vi "Dresden Edit Recipe(in).vi"() -> ()   [LabVIEW 2009] (continued)
                    n653 = local read "R Single DC Step9 Coating Power"() -> (w1514:dbl)
                    n654 = local read "R Single DC Interval length9"() -> (w1513:dbl)
                    n655 = Equal To 0?(x=w1514) -> (x = 0?=w1516:bool)
                    n656 = Equal To 0?(x=w1513) -> (x = 0?=w1515:bool)
                  }
                }
                n657 = case shown="True" w1333 {
                  tunnel: [FALSE w1654] -> w1271
                  tunnel: [FALSE w1651] -> w1270
                  frame #0 {
                  }
                  frame #1 {
                    # "15"
                    # "14"
                    n658 = local read "R Single DC Step4 Coating Power"() -> (w1653:dbl)
                    n659 = local read "R Single DC Interval length4"() -> (w1652:dbl)
                    n660 = Equal To 0?(x=w1653) -> (x = 0?=w1654:bool)
                    n661 = Equal To 0?(x=w1652) -> (x = 0?=w1651:bool)
                  }
                }
                n662 = case shown="True" w1302 {
                  tunnel: [FALSE w1533] -> w1267
                  tunnel: [FALSE w1531] -> w1266
                  frame #0 {
                  }
                  frame #1 {
                    # "19"
                    # "18"
                    n663 = local read "R Single DC Step6 Coating Power"() -> (w1534:dbl)
                    n664 = local read "R Single DC Interval length6"() -> (w1532:dbl)
                    n665 = Equal To 0?(x=w1534) -> (x = 0?=w1533:bool)
                    n666 = Equal To 0?(x=w1532) -> (x = 0?=w1531:bool)
                  }
                }
                n667 = case shown="True" w1326 {
                  tunnel: [FALSE w1628] -> w1251
                  tunnel: [FALSE w1625] -> w1250
                  frame #0 {
                  }
                  frame #1 {
                    # "32"
                    # "31"
                    n668 = local read "R Single RF  Step1 Coating Power"() -> (w1627:dbl)
                    n669 = local read "R Single RF Interval length"() -> (w1626:dbl)
                    n670 = Equal To 0?(x=w1626) -> (x = 0?=w1625:bool)
                    n671 = Equal To 0?(x=w1627) -> (x = 0?=w1628:bool)
                  }
                }
                n672 = case shown="True" w1325 {
                  tunnel: [FALSE w1622] -> w1249
                  tunnel: [FALSE w1619] -> w1248
                  frame #0 {
                  }
                  frame #1 {
                    # "34"
                    # "33"
                    n673 = local read "R Single RF Step2 Coating Power"() -> (w1621:dbl)
                    n674 = local read "R Single RF Interval length2"() -> (w1620:dbl)
                    n675 = Equal To 0?(x=w1621) -> (x = 0?=w1622:bool)
                    n676 = Equal To 0?(x=w1620) -> (x = 0?=w1619:bool)
                  }
                }
                n677 = case shown="True" w1308 {
                  tunnel: [FALSE w1610] -> w1245
                  tunnel: [FALSE w1607] -> w1244
                  frame #0 {
                  }
                  frame #1 {
                    # "38"
                    # "37"
                    n678 = local read "R Single RF Step4 Coating Power"() -> (w1609:dbl)
                    n679 = local read "R Single RF Interval length4"() -> (w1608:dbl)
                    n680 = Equal To 0?(x=w1609) -> (x = 0?=w1610:bool)
                    n681 = Equal To 0?(x=w1608) -> (x = 0?=w1607:bool)
                  }
                }
                n682 = case shown="True" w1298 {
                  tunnel: [FALSE w1502] -> w1241
                  tunnel: [FALSE w1501] -> w1240
                  frame #0 {
                  }
                  frame #1 {
                    # "42"
                    # "41"
                    n683 = local read "R Single RF Step6 Coating Power"() -> (w1504:dbl)
                    n684 = local read "R Single RF Interval length6"() -> (w1503:dbl)
                    n685 = Equal To 0?(x=w1504) -> (x = 0?=w1502:bool)
                    n686 = Equal To 0?(x=w1503) -> (x = 0?=w1501:bool)
                  }
                }
                n687 = case shown="True" w1297 {
                  tunnel: [FALSE w1496] -> w1239
                  tunnel: [FALSE w1495] -> w1237
                  frame #0 {
                  }
                  frame #1 {
                    # "44"
                    # "43"
                    n688 = local read "R Single RF Step7 Coating Power"() -> (w1498:dbl)
                    n689 = local read "R Single RF Interval length7"() -> (w1497:dbl)
                    n690 = Equal To 0?(x=w1498) -> (x = 0?=w1496:bool)
                    n691 = Equal To 0?(x=w1497) -> (x = 0?=w1495:bool)
                  }
                }
                n692 = case shown="True" w1296 {
                  tunnel: [FALSE w1490] -> w1238
                  tunnel: [FALSE w1489] -> _
                  frame #0 {
                  }
                  frame #1 {
                    # "46"
                    # "45"
                    n693 = local read "R Single RF Step8 Coating Power"() -> (w1492:dbl)
                    n694 = local read "R Single RF Interval length8"() -> (w1491:dbl)
                    n695 = Equal To 0?(x=w1492) -> (x = 0?=w1490:bool)
                    n696 = Equal To 0?(x=w1491) -> (x = 0?=w1489:bool)
                  }
                }
                n697 = case shown="True" w1336 {
                  tunnel: [FALSE w1672] -> w1277
                  tunnel: [FALSE w1669] -> w1276
                  frame #0 {
                  }
                  frame #1 {
                    # "9"
                    # "8"
                    n698 = local read "R Single DC Step1 Coating Power"() -> (w1671:dbl)
                    n699 = local read "R Single DC Interval length1"() -> (w1670:dbl)
                    n700 = Equal To 0?(x=w1671) -> (x = 0?=w1672:bool)
                    n701 = Equal To 0?(x=w1670) -> (x = 0?=w1669:bool)
                  }
                }
                n702 = case shown="True" w1335 {
                  tunnel: [FALSE w1666] -> w1275
                  tunnel: [FALSE w1663] -> w1274
                  frame #0 {
                  }
                  frame #1 {
                    # "11"
                    # "10"
                    n703 = local read "R Single DC Step2 Coating Power"() -> (w1665:dbl)
                    n704 = local read "R Single DC Interval length2"() -> (w1664:dbl)
                    n705 = Equal To 0?(x=w1664) -> (x = 0?=w1663:bool)
                    n706 = Equal To 0?(x=w1665) -> (x = 0?=w1666:bool)
                  }
                }
                n707 = case shown="True" w1300 {
                  tunnel: [FALSE w1520] -> w1263
                  tunnel: [FALSE w1519] -> w1262
                  frame #0 {
                  }
                  frame #1 {
                    # "23"
                    # "22"
                    n708 = local read "R Single DC Step8 Coating Power"() -> (w1522:dbl)
                    n709 = local read "R Single DC Interval length8"() -> (w1521:dbl)
                    n710 = Equal To 0?(x=w1522) -> (x = 0?=w1520:bool)
                    n711 = Equal To 0?(x=w1521) -> (x = 0?=w1519:bool)
                  }
                }
                n712 = case shown="True" w1324 {
                  tunnel: [FALSE w1604] -> w1243
                  tunnel: [FALSE w1601] -> w1242
                  frame #0 {
                  }
                  frame #1 {
                    # "40"
                    # "39"
                    n713 = local read "R Single RF Step5 Coating Power"() -> (w1603:dbl)
                    n714 = local read "R Single RF Interval length5"() -> (w1602:dbl)
                    n715 = Equal To 0?(x=w1603) -> (x = 0?=w1604:bool)
                    n716 = Equal To 0?(x=w1602) -> (x = 0?=w1601:bool)
                  }
                }
                n717 = case shown="True" w1334 {
                  tunnel: [FALSE w1660] -> w1273
                  tunnel: [FALSE w1658] -> w1272
                  frame #0 {
                  }
                  frame #1 {
                    # "13"
                    # "12"
                    n718 = local read "R Single DC Step3 Coating Power"() -> (w1659:dbl)
                    n719 = local read "R Single DC Interval length3"() -> (w1657:dbl)
                    n720 = Equal To 0?(x=w1659) -> (x = 0?=w1660:bool)
                    n721 = Equal To 0?(x=w1657) -> (x = 0?=w1658:bool)
                  }
                }
                n722 = case shown="True" w1301 {
                  tunnel: [FALSE w1528] -> w1265
                  tunnel: [FALSE w1527] -> w1264
                  frame #0 {
                  }
                  frame #1 {
                    # "21"
                    # "20"
                    n723 = local read "R Single DC Step7 Coating Power"() -> (w1526:dbl)
                    n724 = local read "R Single DC Interval length7"() -> (w1525:dbl)
                    n725 = Equal To 0?(x=w1526) -> (x = 0?=w1528:bool)
                    n726 = Equal To 0?(x=w1525) -> (x = 0?=w1527:bool)
                  }
                }
                n727 = case shown="True" w1309 {
                  tunnel: [FALSE w1616] -> w1247
                  tunnel: [FALSE w1613] -> w1246
                  frame #0 {
                  }
                  frame #1 {
                    # "36"
                    # "35"
                    n728 = local read "R Single RF Step3 Coating Power"() -> (w1615:dbl)
                    n729 = local read "R Single RF Interval length3"() -> (w1614:dbl)
                    n730 = Equal To 0?(x=w1614) -> (x = 0?=w1613:bool)
                    n731 = Equal To 0?(x=w1615) -> (x = 0?=w1616:bool)
                  }
                }
                n732 = case shown="True" w1327 {
                  tunnel: [FALSE w1631] -> w1252
                  frame #0 {
                  }
                  frame #1 {
                    # "30"
                    n733 = local read "R Single RF Ramp up Time"() -> (w1630:dbl)
                    n734 = Equal To 0?(x=w1630) -> (x = 0?=w1631:bool)
                  }
                }
                n735 = case shown="True" w1179 {
                  tunnel: [FALSE w1508] -> w1259
                  tunnel: [FALSE w1507] -> w1258
                  frame #0 {
                  }
                  frame #1 {
                    # "27"
                    # "26"
                    n736 = local read "R Single DC Step10 Coating Power"() -> (w1510:dbl)
                    n737 = local read "R Single DC Interval length10"() -> (w1509:dbl)
                    n738 = Equal To 0?(x=w1510) -> (x = 0?=w1508:bool)
                    n739 = Equal To 0?(x=w1509) -> (x = 0?=w1507:bool)
                  }
                }
                n740 = case shown="True" w1331 {
                  tunnel: [FALSE w1638] -> w1257
                  tunnel: [FALSE w1634] -> w1256
                  frame #0 {
                  }
                  frame #1 {
                    # "29"
                    # "28"
                    n741 = local read "R Single RF Target material"() -> (w1636:string)
                    n742 = local read "Power_single_rf_list_open"() -> (w1635:bool)
                    n743 = Not(x=w1635) -> (.not. x?=w1634:bool)
                    n744 = Equal?(x=w1636, y="") -> (x = y?=w1638:bool)
                  }
                }
                n745 = case shown="True" w1341 {
                  tunnel: [FALSE w1688] -> w1317
                  tunnel: [FALSE w1686] -> w1316
                  frame #0 {
                  }
                  frame #1 {
                    # "4"
                    # "3"
                    n746 = local read "R_Single Microwave Power"() -> (w1689:dbl)
                    n747 = local read "R Single Pass Number"() -> (w1687:dbl)
                    n748 = Equal To 0?(x=w1689) -> (x = 0?=w1688:bool)
                    n749 = Equal To 0?(x=w1687) -> (x = 0?=w1686:bool)
                  }
                }
                n750 = case shown="True" w1303 {
                  tunnel: [FALSE w1536] -> w1307
                  frame #0 {
                  }
                  frame #1 {
                    # "5"
                    n751 = local read "R_Single Microwave Time"() -> (w1537:dbl)
                    n752 = Equal To 0?(x=w1537) -> (x = 0?=w1536:bool)
                  }
                }
                n753 = case shown="True" w1337 {
                  tunnel: [FALSE w1678] -> w1315
                  tunnel: [FALSE ("Power_singledc_list_open") w1675] -> w1278
                  frame #0 {
                    (unwired) FALSE
                  }
                  frame #1 {
                    # "7"
                    # "6"
                    n754 = local read "R Single DC Target material"() -> (w1679:string)
                    n755 = local read "Power_singledc_list_open"() -> (w1676:bool)
                    n756 = Not(x=w1676) -> (.not. x?=w1675:bool)
                    n757 = Equal?(x=w1679, y="") -> (x = y?=w1678:bool)
                  }
                }
                n758 = local read "R_Recipe_type_selection"() -> (w1282:enum32{"Single Recipe", "Combination Sputter"})
                n759 = local read "R_Recipe_type_selection"() -> (w1163:enum32{"Single Recipe", "Combination Sputter"})
                n760 = Equal?(x=w1282, y=0) -> (x = y?=w1280:bool)
                n761 = case shown="True" w1280 {
                  tunnel: [FALSE w1400] -> w1177
                  frame #0 {
                  }
                  frame #1 {
                    n762 = local read "R_Simple_Coating Type Selection"() -> (w1401:T2)
                    n763 = Equal?(x=w1401, y=1) -> (x = y?=w1400:bool)
                  }
                }
                n764 = local read "R_Web_selection"() -> (w1166:enum32{"Web", "Other"})
                n765 = local read "R_Web_selection"() -> (w1346:enum32{"Web", "Other"})
                n766 = local read "Web_selection_tab"() -> (w1175:T4)
                n767 = local read "Web_selection_tab"() -> (w1173:T4)
                n768 = Equal?(x=w1166, y=0) -> (x = y?=w1165:bool)
                n769 = Equal?(x=w1163, y=0) -> (x = y?=w1164:bool)
                n770 = Equal?(x=w1346, y=0) -> (x = y?=w1170:bool)
                n771 = case shown="True" w1164 {
                  tunnel: [FALSE w1367] -> w1168
                  frame #0 {
                  }
                  frame #1 {
                    n772 = local read "R_Web_selection"() -> (w1366:enum32{"Web", "Other"})
                    n773 = Equal?(x=w1366, y=0) -> (x = y?=w1367:bool)
                  }
                }
                n774 = Equal?(x=w1175, y=0) -> (x = y?=w1174:bool)
                n775 = Equal?(x=w1173, y=0) -> (x = y?=w1171:bool)
                n776 = local read "R_Web_selection"() -> (w1311:enum32{"Web", "Other"})
                n777 = local read "R Single RF Step9 Coating Power Active"() -> (w1295:bool)
                n778 = case shown="True" w1170 {
                  tunnel: [FALSE w1374] -> w1188
                  tunnel: [FALSE w1373] -> w1187
                  frame #0 {
                  }
                  frame #1 {
                    # "96"
                    # "95"
                    n779 = local read "R Maximum diameter"() -> (w1371:dbl)
                    n780 = local read "R Minimum diameter"() -> (w1372:dbl)
                    n781 = Equal To 0?(x=w1372) -> (x = 0?=w1374:bool)
                    n782 = Equal To 0?(x=w1371) -> (x = 0?=w1373:bool)
                  }
                }
                n783 = local read "R Single RF Step10 Coating Power Active"() -> (w1294:bool)
                n784 = local read "R Cmb Step1 Coating Power Active"() -> (w1292:bool)
                n785 = local read "R Cmb Step4 Coating Power Active"() -> (w1289:bool)
                n786 = local read "R Cmb Step3 Coating Power Active"() -> (w1290:bool)
                n787 = local read "R Cmb Step2 Coating Power Active"() -> (w1291:bool)
                n788 = local read "R Cmb Step5 Coating Power Active"() -> (w1288:bool)
                n789 = local read "R Cmb Step7 Coating Power Active"() -> (w1286:bool)
                n790 = local read "R Cmb Step6 Coating Power Active"() -> (w1287:bool)
                n791 = local read "R Cmb Step10 Coating Power Active"() -> (w1283:bool)
                n792 = local read "R Cmb Step8 Coating Power Active"() -> (w1285:bool)
                n793 = local read "R_Recipe_type_selection"() -> (w1293:enum32{"Single Recipe", "Combination Sputter"})
                n794 = local read "R Cmb Step9 Coating Power Active"() -> (w1284:bool)
                n795 = case shown="True" w1174 {
                  tunnel: [FALSE w1382] -> w1180
                  frame #0 {
                  }
                  frame #1 {
                    n796 = local read "R_Simple_Coating Type Selection"() -> (w1380:T2)
                    n797 = Equal?(x=w1380, y=2) -> (x = y?=w1382:bool)
                  }
                }
                n798 = case shown="False" w1171 {
                  tunnel: [FALSE w1376] -> w1279
                  frame #0 {
                  }
                  frame #1 {
                    n799 = local read "R_Recipe_type_selection"() -> (w1378:enum32{"Single Recipe", "Combination Sputter"})
                    n800 = Equal?(x=w1378, y=1) -> (x = y?=w1376:bool)
                  }
                }
                n801 = case shown="True" w1177 {
                  tunnel: [FALSE w1384] -> w1178
                  frame #0 {
                  }
                  frame #1 {
                    n802 = local read "Web_selection_tab"() -> (w1385:T4)
                    n803 = Equal?(x=w1385, y=0) -> (x = y?=w1384:bool)
                  }
                }
                n804 = local read "R Single RF Ramp down"() -> (w1323:bool)
                n805 = local read "Thickness_Monitor_Active"() -> (w1320:bool)
                n806 = Equal?(x=w1311, y=1) -> (x = y?=w1313:bool)
                n807 = case shown="True" w1313 {
                  tunnel: [FALSE w1545] -> w1190
                  tunnel: [FALSE w1544] -> w1189
                  frame #0 {
                  }
                  frame #1 {
                    # "94"
                    # "93"
                    n808 = local read "R_Thickness Selection"() -> (w1551:enum32{"Thickness", "Time"})
                    n809 = local read "R_Thickness Selection"() -> (w1548:enum32{"Thickness", "Time"})
                    n810 = Equal?(x=w1551, y=0) -> (x = y?=w1547:bool)
                    n811 = Equal?(x=w1548, y=1) -> (x = y?=w1546:bool)
                    n812 = case shown="True" w1547 {
                      tunnel: [FALSE w1556] -> w1545
                      frame #0 {
                      }
                      frame #1 {
                        n813 = local read "R_Target Thickness Value"() -> (w1557:dbl)
                        n814 = Equal To 0?(x=w1557) -> (x = 0?=w1556:bool)
                      }
                    }
                    n815 = case shown="True" w1546 {
                      tunnel: [FALSE w1553] -> w1544
                      frame #0 {
                      }
                      frame #1 {
                        n816 = local read "R_Duration"() -> (w1554:dbl)
                        n817 = Equal To 0?(x=w1554) -> (x = 0?=w1553:bool)
                      }
                    }
                  }
                }
                n818 = case shown="True" w1168 {
                  tunnel: [FALSE w1364] -> w1186
                  frame #0 {
                  }
                  frame #1 {
                    # "97"
                    n819 = local read "R Web speed(cm/min)"() -> (w1363:dbl)
                    n820 = Equal To 0?(x=w1363) -> (x = 0?=w1364:bool)
                  }
                }
                n821 = case shown="True" w1165 {
                  tunnel: [FALSE w1361] -> w1185
                  tunnel: [FALSE w1360] -> w1184
                  tunnel: [FALSE w1359] -> w1162
                  frame #0 {
                  }
                  frame #1 {
                    # "100"
                    # "99"
                    # "98"
                    n822 = local read "R Web thickness"() -> (w1356:dbl)
                    n823 = local read "R Tension Value"() -> (w1358:dbl)
                    n824 = local read "R  Total length"() -> (w1357:dbl)
                    n825 = Equal To 0?(x=w1356) -> (x = 0?=w1361:bool)
                    n826 = Equal To 0?(x=w1358) -> (x = 0?=w1360:bool)
                    n827 = Equal To 0?(x=w1357) -> (x = 0?=w1359:bool)
                  }
                }
                n828 = Equal?(x=w1293, y=1) -> (x = y?=w1321:bool)
                n829 = case shown="True" w1285 {
                  tunnel: [FALSE w1429] -> w1204
                  tunnel: [FALSE w1428] -> w1203
                  tunnel: [FALSE w1427] -> w1202
                  frame #0 {
                  }
                  frame #1 {
                    # "81"
                    # "80"
                    # "79"
                    n830 = local read "R Cmb Ch2 Step8 Coating Power"() -> (w1426:dbl)
                    n831 = local read "R Cmb Ch3 Step8 Coating Power"() -> (w1425:dbl)
                    n832 = local read "R Cmb Interval length 8"() -> (w1424:dbl)
                    n833 = Equal To 0?(x=w1426) -> (x = 0?=w1429:bool)
                    n834 = Equal To 0?(x=w1425) -> (x = 0?=w1428:bool)
                    n835 = Equal To 0?(x=w1424) -> (x = 0?=w1427:bool)
                  }
                }
                n836 = case shown="True" w1321 {
                  tunnel: [FALSE w1591] -> w1231
                  tunnel: [FALSE w1590] -> w1229
                  tunnel: [FALSE w1587] -> w1230
                  tunnel: [FALSE w1586] -> w1228
                  tunnel: [FALSE w1584] -> w1226
                  tunnel: [FALSE ("Power_list_open") w1582] -> w1227
                  frame #0 {
                  }
                  frame #1 {
                    # "57"
                    # "56"
                    # "55"
                    # "54"
                    # "53"
                    # "52"
                    n837 = local read "R Cmb Ch2 Target material"() -> (w1594:string)
                    n838 = local read "R Cmb Ch3 Target material"() -> (w1592:string)
                    n839 = local read "R Cmb Number of cycle"() -> (w1585:dbl)
                    n840 = local read "R_Cmb_Ch2_Web_speed"() -> (w1589:dbl)
                    n841 = local read "R_Cmb_Ch3_Web_speed"() -> (w1588:dbl)
                    n842 = local read "Power_list_open_multi"() -> (w1583:bool)
                    n843 = Equal?(x=w1592, y="") -> (x = y?=w1590:bool)
                    n844 = Equal?(x=w1594, y="") -> (x = y?=w1591:bool)
                    n845 = Equal To 0?(x=w1589) -> (x = 0?=w1587:bool)
                    n846 = Equal To 0?(x=w1588) -> (x = 0?=w1586:bool)
                    n847 = Equal To 0?(x=w1585) -> (x = 0?=w1584:bool)
                    n848 = Not(x=w1583) -> (.not. x?=w1582:bool)
                  }
                }
                n849 = case shown="True" w1295 {
                  tunnel: [FALSE w1485] -> w1236
                  tunnel: [FALSE w1483] -> w1235
                  frame #0 {
                  }
                  frame #1 {
                    # "48"
                    # "47"
                    n850 = local read "R Single RF Step9 Coating Power"() -> (w1486:dbl)
                    n851 = local read "R Single RF Interval length9"() -> (w1484:dbl)
                    n852 = Equal To 0?(x=w1484) -> (x = 0?=w1483:bool)
                    n853 = Equal To 0?(x=w1486) -> (x = 0?=w1485:bool)
                  }
                }
                n854 = case shown="True" w1294 {
                  tunnel: [FALSE w1478] -> w1234
                  tunnel: [FALSE w1477] -> w1233
                  frame #0 {
                  }
                  frame #1 {
                    # "50"
                    # "49"
                    n855 = local read "R Single RF Step10 Coating Power"() -> (w1480:dbl)
                    n856 = local read "R Single RF Interval length10"() -> (w1479:dbl)
                    n857 = Equal To 0?(x=w1479) -> (x = 0?=w1477:bool)
                    n858 = Equal To 0?(x=w1480) -> (x = 0?=w1478:bool)
                  }
                }
                n859 = case shown="True" w1323 {
                  tunnel: [FALSE w1597] -> w1232
                  frame #0 {
                  }
                  frame #1 {
                    # "51"
                    n860 = local read "R Single RF Ramp down Time"() -> (w1598:dbl)
                    n861 = Equal To 0?(x=w1598) -> (x = 0?=w1597:bool)
                  }
                }
                n862 = case shown="True" w1283 {
                  tunnel: [FALSE w1411] -> w1198
                  tunnel: [FALSE w1410] -> w1197
                  tunnel: [FALSE w1409] -> w1196
                  frame #0 {
                  }
                  frame #1 {
                    # "87"
                    # "86"
                    # "85"
                    n863 = local read "R Cmb Ch2 Step10 Coating Power"() -> (w1408:dbl)
                    n864 = local read "R Cmb Ch3 Step10 Coating Power"() -> (w1407:dbl)
                    n865 = local read "R Cmb Interval length 10"() -> (w1406:dbl)
                    n866 = Equal To 0?(x=w1408) -> (x = 0?=w1411:bool)
                    n867 = Equal To 0?(x=w1407) -> (x = 0?=w1410:bool)
                    n868 = Equal To 0?(x=w1406) -> (x = 0?=w1409:bool)
                  }
                }
                n869 = case shown="True" w1287 {
                  tunnel: [FALSE w1447] -> w1210
                  tunnel: [FALSE w1446] -> w1209
                  tunnel: [FALSE w1445] -> w1208
                  frame #0 {
                  }
                  frame #1 {
                    # "75"
                    # "74"
                    # "73"
                    n870 = local read "R Cmb Ch2 Step6 Coating Power"() -> (w1444:dbl)
                    n871 = local read "R Cmb Ch3 Step6 Coating Power"() -> (w1443:dbl)
                    n872 = local read "R Cmb Interval length 6"() -> (w1442:dbl)
                    n873 = Equal To 0?(x=w1444) -> (x = 0?=w1447:bool)
                    n874 = Equal To 0?(x=w1443) -> (x = 0?=w1446:bool)
                    n875 = Equal To 0?(x=w1442) -> (x = 0?=w1445:bool)
                  }
                }
                n876 = case shown="True" w1284 {
                  tunnel: [FALSE w1420] -> w1201
                  tunnel: [FALSE w1419] -> w1200
                  tunnel: [FALSE w1418] -> w1199
                  frame #0 {
                  }
                  frame #1 {
                    # "84"
                    # "83"
                    # "82"
                    n877 = local read "R Cmb Ch2 Step9 Coating Power"() -> (w1417:dbl)
                    n878 = local read "R Cmb Ch3 Step9 Coating Power"() -> (w1416:dbl)
                    n879 = local read "R Cmb Interval length 9"() -> (w1415:dbl)
                    n880 = Equal To 0?(x=w1417) -> (x = 0?=w1420:bool)
                    n881 = Equal To 0?(x=w1416) -> (x = 0?=w1419:bool)
                    n882 = Equal To 0?(x=w1415) -> (x = 0?=w1418:bool)
                  }
                }
                n883 = case shown="True" w1286 {
                  tunnel: [FALSE w1438] -> w1207
                  tunnel: [FALSE w1437] -> w1206
                  tunnel: [FALSE w1436] -> w1205
                  frame #0 {
                  }
                  frame #1 {
                    # "78"
                    # "77"
                    # "76"
                    n884 = local read "R Cmb Ch2 Step7 Coating Power"() -> (w1435:dbl)
                    n885 = local read "R Cmb Ch3 Step7 Coating Power"() -> (w1434:dbl)
                    n886 = local read "R Cmb Interval length 7"() -> (w1433:dbl)
                    n887 = Equal To 0?(x=w1435) -> (x = 0?=w1438:bool)
                    n888 = Equal To 0?(x=w1434) -> (x = 0?=w1437:bool)
                    n889 = Equal To 0?(x=w1433) -> (x = 0?=w1436:bool)
                  }
                }
                n890 = case shown="True" w1292 {
                  tunnel: [FALSE w1575] -> w1225
                  tunnel: [FALSE w1574] -> w1224
                  tunnel: [FALSE w1573] -> w1223
                  frame #0 {
                  }
                  frame #1 {
                    # "60"
                    # "59"
                    # "58"
                    n891 = local read "R Cmb Ch2 Step1 Coating Power"() -> (w1571:dbl)
                    n892 = local read "R Cmb Ch3 Step1 Coating Power"() -> (w1570:dbl)
                    n893 = local read "R Cmb Interval length 1"() -> (w1572:dbl)
                    n894 = Equal To 0?(x=w1571) -> (x = 0?=w1575:bool)
                    n895 = Equal To 0?(x=w1570) -> (x = 0?=w1574:bool)
                    n896 = Equal To 0?(x=w1572) -> (x = 0?=w1573:bool)
                  }
                }
                n897 = case shown="True" w1291 {
                  tunnel: [FALSE w1566] -> w1222
                  tunnel: [FALSE w1565] -> w1221
                  tunnel: [FALSE w1564] -> w1220
                  frame #0 {
                  }
                  frame #1 {
                    # "63"
                    # "62"
                    # "61"
                    n898 = local read "R Cmb Ch2 Step2 Coating Power"() -> (w1563:dbl)
                    n899 = local read "R Cmb Ch3 Step2 Coating Power"() -> (w1562:dbl)
                    n900 = local read "R Cmb Interval length 2"() -> (w1561:dbl)
                    n901 = Equal To 0?(x=w1563) -> (x = 0?=w1566:bool)
                    n902 = Equal To 0?(x=w1562) -> (x = 0?=w1565:bool)
                    n903 = Equal To 0?(x=w1561) -> (x = 0?=w1564:bool)
                  }
                }
                n904 = case shown="True" w1290 {
                  tunnel: [FALSE w1474] -> w1219
                  tunnel: [FALSE w1473] -> w1218
                  tunnel: [FALSE w1472] -> w1217
                  frame #0 {
                  }
                  frame #1 {
                    # "66"
                    # "65"
                    # "64"
                    n905 = local read "R Cmb Ch3 Step3 Coating Power"() -> (w1470:dbl)
                    n906 = local read "R Cmb Ch2 Step3 Coating Power"() -> (w1471:dbl)
                    n907 = local read "R Cmb Interval length 3"() -> (w1469:dbl)
                    n908 = Equal To 0?(x=w1471) -> (x = 0?=w1474:bool)
                    n909 = Equal To 0?(x=w1470) -> (x = 0?=w1473:bool)
                    n910 = Equal To 0?(x=w1469) -> (x = 0?=w1472:bool)
                  }
                }
                n911 = case shown="True" w1289 {
                  tunnel: [FALSE w1465] -> w1216
                  tunnel: [FALSE w1464] -> w1215
                  tunnel: [FALSE w1463] -> w1214
                  frame #0 {
                  }
                  frame #1 {
                    # "69"
                    # "68"
                    # "67"
                    n912 = local read "R Cmb Ch3 Step4 Coating Power"() -> (w1461:dbl)
                    n913 = local read "R Cmb Ch2 Step4 Coating Power"() -> (w1462:dbl)
                    n914 = local read "R Cmb Interval length 4"() -> (w1460:dbl)
                    n915 = Equal To 0?(x=w1462) -> (x = 0?=w1465:bool)
                    n916 = Equal To 0?(x=w1461) -> (x = 0?=w1464:bool)
                    n917 = Equal To 0?(x=w1460) -> (x = 0?=w1463:bool)
                  }
                }
                n918 = case shown="True" w1288 {
                  tunnel: [FALSE w1456] -> w1213
                  tunnel: [FALSE w1455] -> w1212
                  tunnel: [FALSE w1454] -> w1211
                  frame #0 {
                  }
                  frame #1 {
                    # "72"
                    # "71"
                    # "70"
                    n919 = local read "R Cmb Ch2 Step5 Coating Power"() -> (w1453:dbl)
                    n920 = local read "R Cmb Ch3 Step5 Coating Power"() -> (w1452:dbl)
                    n921 = local read "R Cmb Interval length 5"() -> (w1451:dbl)
                    n922 = Equal To 0?(x=w1453) -> (x = 0?=w1456:bool)
                    n923 = Equal To 0?(x=w1452) -> (x = 0?=w1455:bool)
                    n924 = Equal To 0?(x=w1451) -> (x = 0?=w1454:bool)
                  }
                }
                n925 = case shown="True" w1320 {
                  tunnel: [FALSE w1700] -> w1195
                  tunnel: [FALSE w1699] -> w1194
                  tunnel: [FALSE w1697] -> w1193
                  frame #0 {
                  }
                  frame #1 {
                    # "90"
                    # "89"
                    # "88"
                    n926 = local read "R Toooling_factor"() -> (w1698:dbl)
                    n927 = local read "R Material_density"() -> (w1702:dbl)
